vi "EG_G5210 CheckStatus.vi"(6 "ShowStatMess":bool=TRUE caption="Show Status Message", 7 "StatusByteRef":refnum<vi>, 8 "error in (no error)":errorcluster, 9 "Ask Correction":bool, 10 "Autoscale":bool, 11 "Ressource VISA In":refnum<visa-resource-name>="GPIB0::8::INSTR") -> (0 "error out":errorcluster, 1 "Warning":bool, 2 "Ask Correction Out":bool, 3 "Ressource VISA Out":refnum<visa-resource-name>="GPIB0::8::INSTR", 4 "Reprise":bool, 5 "Status Byte":bool[](array[boolean]))   [LabVIEW 2019]
uses:
  <userlib>/EG_G 5210 LIA/CheckStatusState.ctl
  <userlib>/GenProg/WritebyWeakRefNum.vi
panel:
  # "Command Complete"
  # "Command Par Error"
  # "Pll unlck"
  # "New Val Avail"
  # "SRQ Asserted"
  # "Data Available"
  # "Invalid Command"
  # "Overload"
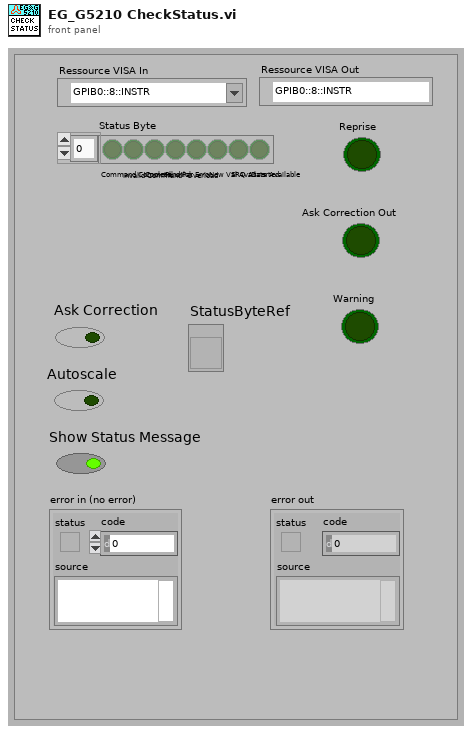
[diagram p1: front panel]
types:
  T1 = typedef "CheckStatusState.ctl" = enum16{"Read Status", "Status Message", "Find Error", "PLL", "Overload", "Change Scale"}
  T2 = enum32{"Invalid", "Standard", "Closed", "Hidden", "Minimized", "Maximized"}
  T3 = enum16{"Left Button", "Center Button", "Right Button", "Window Close"}
  T4 = enum32{"Bad", "Idle", "Run top level", "Running"}
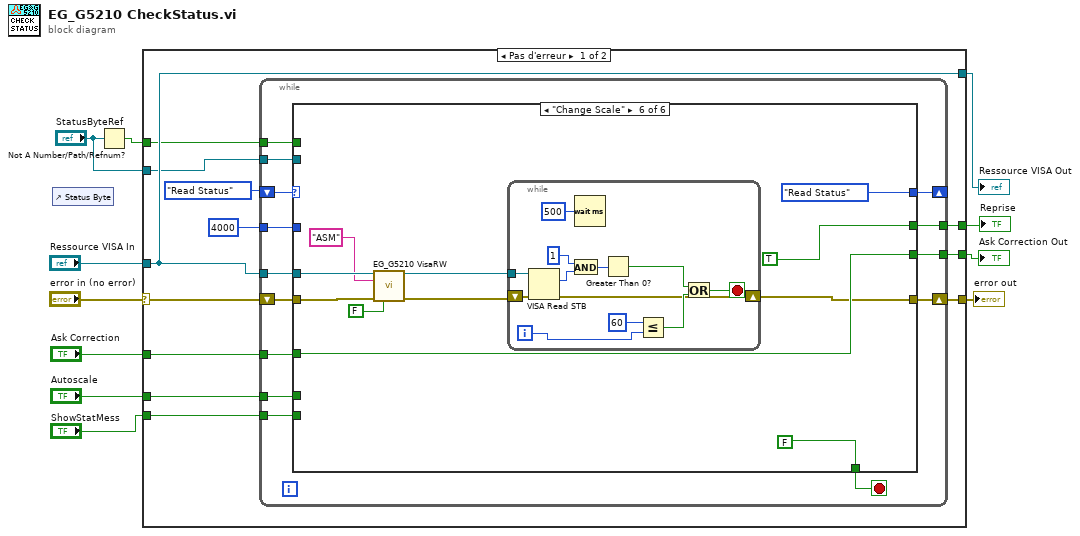
[diagram p0: block diagram]
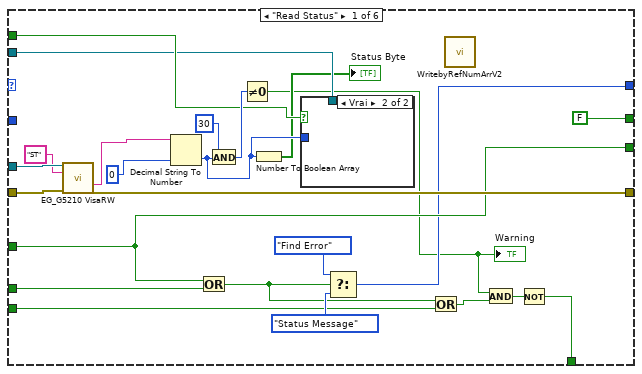
[diagram p2: hidden frame]
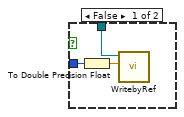
[diagram p3: hidden frame]
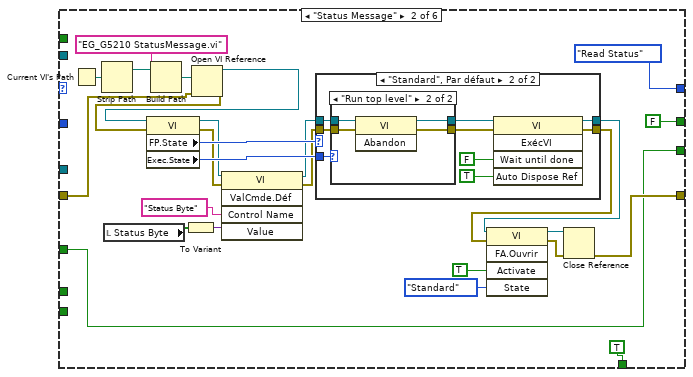
[diagram p4: hidden frame]
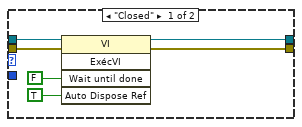
[diagram p5: hidden frame]
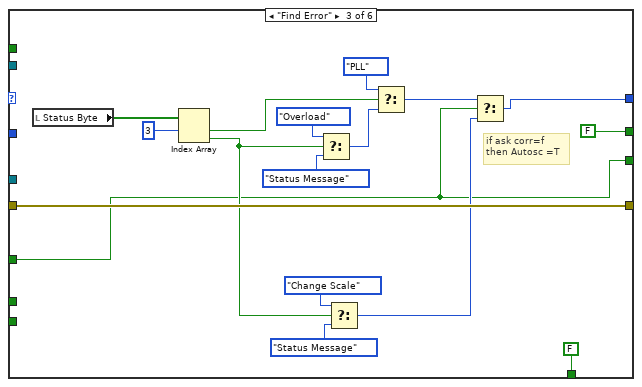
[diagram p7: hidden frame]
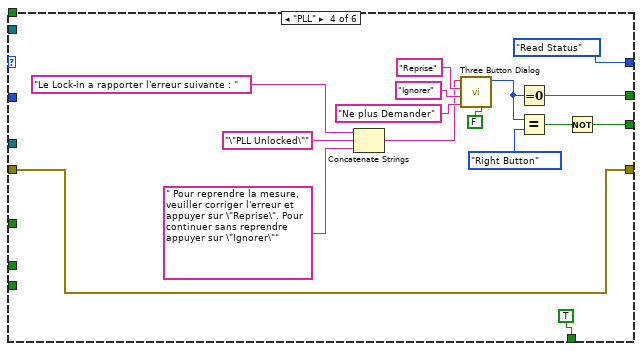
[diagram p8: hidden frame]
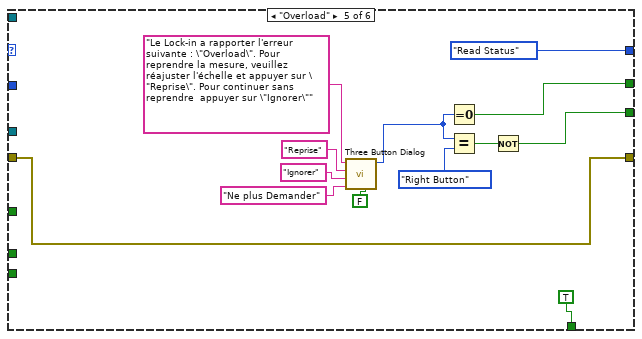
[diagram p9: hidden frame]
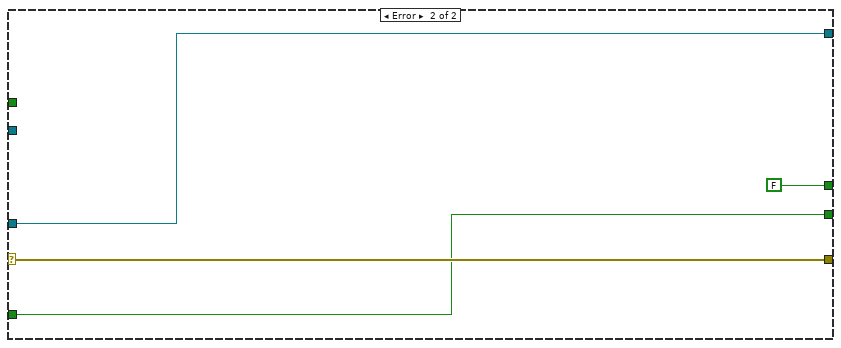
[diagram p10: hidden frame]
diagram:
  n1 = control-ref of="Status Byte"() -> ()  [unwired: 1 out]
  n2 = Not A Number/Path/Refnum?(number/path/refnum="StatusByteRef") -> (NaN/Path/Refnum?=w3:bool)
  n3 = case shown="Pas d'erreur" "error in (no error)" {
    selector: "error in (no error)" -> [w19 w185]
    tunnel: [w22 w185] -> w10
    tunnel: "Autoscale" -> [w21 _]
    tunnel: "Ask Correction" -> [w20 w183]
    tunnel: [w18 FALSE] -> w6
    tunnel: [w17 w183] -> w7
    tunnel: "Ressource VISA In" -> [w16 w182]
    tunnel: [w16 w182] -> w4
    tunnel: w3 -> [w14 _]
    tunnel: "StatusByteRef" -> [w13 _]
    tunnel: "ShowStatMess" -> [w12 _]
    frame No Error {
      n4 = while {
        shift-right: [w32] -> _
        shift-left: CheckStatusState."Read Status" ("Énum") -> [w37]
        shift-right: [w35] -> w22
        shift-left: w19 -> [w36]
        tunnel: 4000 ("timeout ms (488.2 global)") -> [w34]
        tunnel: w21 -> [w31]
        tunnel: w20 -> [w30]
        tunnel: w16 -> [w29]
        tunnel: [w28] -> w18
        tunnel: [w27] -> w17
        tunnel: w14 -> [w26]
        tunnel: w13 -> [w25]
        tunnel: w12 -> [w24]
        stop <- w33 stop-if-true
        n5 = case shown="\"Change Scale\"" w37 {
          tunnel: w36 -> [w61 w78 w124 w134 w157 w169]
          tunnel: [w60 w79 w124 w134 w157 w160] -> w35
          tunnel: w34 -> [_ _ _ _ _ _]
          tunnel: [w38 TRUE FALSE TRUE TRUE FALSE] -> w33
          tunnel: [w52 CheckStatusState."Read Status" w118 CheckStatusState."Read Status" CheckStatusState."Read Status" CheckStatusState."Read Status"] -> w32
          tunnel: w31 -> [w53 _ _ _ _ _]
          tunnel: w30 -> [w54 w73 w113 _ _ w168]
          tunnel: w29 -> [w59 _ _ _ _ w166]
          tunnel: [w54 w73 w113 w131 w155 w168] -> w27
          tunnel: [FALSE FALSE FALSE w133 w156 TRUE] -> w28
          tunnel: w26 -> [w47 _ _ _ _ _]
          tunnel: w25 -> [w45 _ _ _ _ _]
          tunnel: w24 -> [w42 _ _ _ _ _]
          frame "Read Status" {
            n6 = call <userlib>:"EG_G5210 VisaRW.vi"("VISA Rsrc"=w59, "ChaineCom"="ST", "error in (no error)"=w61) -> ("ChaineRep"=w51:string, "error out"=w60:errorcluster)  [unwired: 9 in, 2 out]
            n7 = Decimal String To Number(string=w51, default (0L)=u8 0 ("default (0 I32)")) -> (number=w46:u8)  [unwired: 1 in, 1 out]
            n8 = Or(x=w54, y=w53) -> (x .or. y?=w43:bool)
            n9 = And(x=u8 30, y=w46) -> (x .and. y?=w48:u8)
            n10 = Not Equal To 0?(x=w48) -> (x != 0?=w41:bool)
            "Warning" <- w41
            n11 = Number To Boolean Array(number=w46) -> (Boolean array=→"Status Byte":bool[])
            n12 = case shown="Vrai" w47 {
              tunnel: w46 -> [w63 _]
              tunnel: w45 -> [w64 _]
              frame False {
                n13 = To Double Precision Float(number=w63) -> (double precision float=w62:dbl)
                n14 = call-poly <userlib>:"WritebyRef.vi"("Valeur"=w62, "Control Ref"=w64) -> ()  [unwired: 9 in, 1 out]
              }
              frame True {
              }
            }
            n15 = Select(t=CheckStatusState."Find Error", s=w43, f=CheckStatusState."Status Message") -> (s? t:f=w52:T1)
            n16 = Or(x=w43, y=w42) -> (x .or. y?=w40:bool)
            n17 = call <userlib>:"WritebyRefNumArrV2.vi"() -> ()  [unwired: 11 in, 1 out]
            n18 = And(x=w41, y=w40) -> (x .and. y?=w39:bool)
            n19 = Not(x=w39) -> (.not. x?=w38:bool)
          }
          frame "Status Message" {
            n20 = Current VI's Path() -> (path=w89:path)
            n21 = Strip Path(path=w89) -> (stripped path=w90:path)  [unwired: 1 out]
            n22 = local read "Status Byte"() -> (w76:bool[])
            n23 = Build Path(base path=w90, name or relative path="EG_G5210 StatusMessage.vi" ("nom ou chemin relatif")) -> (appended path=w85:path)
            n24 = To Variant(anything=w76) -> (Variant=w82:variant)
            n25 = Open VI Reference(vi path=w85, error in (no error)=w78) -> (vi reference=w86:refnum<vi>, error out=w77:errorcluster)  [unwired: 4 in]
            n26 = property class="VI"(reference=w86, error in=w77) -> (reference out=w66:refnum<vi>, error out=w67:errorcluster, "FP.State"=w87:T2, "Exec.State"=w88:T4)
            n27 = invoke class="VI" method="ValCmde.Déf"(reference=w66, error in=w67, "Control Name"="Status Byte" ("Nom de la commande"), "Value"=w82) -> (reference out=w68:refnum<vi>, error out=w69:errorcluster)  [unwired: 1 in, 3 out]
            n28 = case shown="\"Standard\", Par défaut" w87 {
              tunnel: [w94 w103] -> w70
              tunnel: w68 -> [w95 w101]
              tunnel: w88 -> [_ w102]
              tunnel: w69 -> [w93 w100]
              tunnel: [w92 w98] -> w71
              frame "Closed" {
                n29 = invoke class="VI" method="ExécVI"(reference=w95, error in=w93, "Wait until done"=FALSE ("Attendre la fin"), "Auto Dispose Ref"=TRUE ("Supprimer la référence automatiquement")) -> (reference out=w94:refnum<vi>, error out=w92:errorcluster)  [unwired: 1 in, 3 out]
              }
              frame "Standard", Default {
                n30 = case shown="\"Run top level\"" w102 {
                  tunnel: [w108 w112] -> w104
                  tunnel: w101 -> [w108 w111]
                  tunnel: w100 -> [w107 w110]
                  tunnel: [w107 w109] -> w99
                  frame "Idle", Default {
                  }
                  frame "Run top level" {
                    n31 = invoke class="VI" method="Abandon"(reference=w111, error in=w110) -> (reference out=w112:refnum<vi>, error out=w109:errorcluster)  [unwired: 1 in, 1 out]
                  }
                }
                n32 = invoke class="VI" method="ExécVI"(reference=w104, error in=w99, "Wait until done"=FALSE ("Attendre la fin"), "Auto Dispose Ref"=TRUE ("Supprimer la référence automatiquement")) -> (reference out=w103:refnum<vi>, error out=w98:errorcluster)  [unwired: 1 in, 3 out]
              }
            }
            n33 = invoke class="VI" method="FA.Ouvrir"(reference=w70, error in=w71, "Activate"=TRUE ("Activer ?"), "State"=T2."Standard" ("État")) -> (reference out=w81:refnum<vi>, error out=w80:errorcluster)  [unwired: 1 in, 3 out]
            n34 = Close Reference(reference=w81, error in (no error)=w80) -> (error out=w79:errorcluster)
          }
          frame "Find Error" {
            # "if ask corr=f\nthen Autosc =T"
            n35 = local read "Status Byte"() -> (w128:bool[])
            n36 = Index Array(array=w128, index #1=3 ("indice")) -> (element #1=w115:bool, element #2=w114:bool)  [unwired: 1 in]
            n37 = Select(t=CheckStatusState."Overload", s=w114, f=CheckStatusState."Status Message") -> (s? t:f=w127:T1)
            n38 = Select(t=CheckStatusState."Change Scale", s=w114, f=CheckStatusState."Status Message") -> (s? t:f=w119:T1)
            n39 = Select(t=CheckStatusState."PLL", s=w115, f=w127) -> (s? t:f=w121:T1)
            n40 = Select(t=w121, s=w113, f=w119) -> (s? t:f=w118:T1)
          }
          frame "PLL" {
            n41 = Concatenate Strings("Le Lock-in a rapporter l'erreur suivante : ", "\"PLL Unlocked\"", " Pour reprendre la mesure, veuiller corriger l'erreur et appuyer sur \"Reprise\". Pour continuer sans reprendre  appuyer sur \"Ignorer\"" ("message")) -> (w139:string)
            n42 = call <vilib>:"Three Button Dialog.vi"("Allow user to close window? (TRUE)"=FALSE, "Right Button Text (\"Cancel\")"="Ne plus Demander" ("F button name (\"Cancel\")"), "Center Button Text (\"No\")"="Ignorer" ("F button name (\"Cancel\")"), "Left Button Text (\"Yes\")"="Reprise" ("T button name (\"OK\")"), "message"=w139) -> ("Which Button?"=w137:T3)  [unwired: 6 in]
            n43 = Equal To 0?(x=w137) -> (x = 0?=w133:bool)
            n44 = Equal?(x=w137, y=T3."Right Button") -> (x = y?=w132:bool)
            n45 = Not(x=w132) -> (.not. x?=w131:bool)
          }
          frame "Overload" {
            n46 = call <vilib>:"Three Button Dialog.vi"("Allow user to close window? (TRUE)"=FALSE, "Right Button Text (\"Cancel\")"="Ne plus Demander" ("F button name (\"Cancel\")"), "Center Button Text (\"No\")"="Ignorer" ("F button name (\"Cancel\")"), "Left Button Text (\"Yes\")"="Reprise" ("T button name (\"OK\")"), "message"="Le Lock-in a rapporter l'erreur suivante : \"Overload\". Pour reprendre la mesure, veuillez réajuster l'échelle et appuyer sur \"Reprise\". Pour continuer sans reprendre  appuyer sur \"Ignorer\"") -> ("Which Button?"=w147:T3)  [unwired: 6 in]
            n47 = Equal To 0?(x=w147) -> (x = 0?=w156:bool)
            n48 = Equal?(x=w147, y=T3."Right Button") -> (x = y?=w146:bool)
            n49 = Not(x=w146) -> (.not. x?=w155:bool)
          }
          frame "Change Scale" {
            n50 = call <userlib>:"EG_G5210 VisaRW.vi"("VISA Rsrc"=w166, "ChaineCom"="ASM", "error in (no error)"=w169, "Lecture?(T)"=FALSE) -> ("VISA Rsrc Out"=w162:refnum<visa-resource-name>, "error out"=w159:errorcluster)  [unwired: 8 in, 2 out]
            n51 = while {
              tunnel: w162 -> [w177]
              shift-right: [w171] -> w160
              shift-left: w159 -> [w170]
              i -> [w180]
              stop <- w178 stop-if-true
              n52 = VISA Read STB(8:w170, 11:w177) -> (0:w171:errorcluster, 2:w176:u16)  [unwired: 1 out]
              n53 = And(x=u16 1, y=w176) -> (x .and. y?=w174:u16)
              n54 = Wait (ms)(milliseconds to wait=u32 500 ("attente (ms)")) -> ()  [unwired: 1 out]
              n55 = Greater Than 0?(x=w174) -> (x > 0?=w172:bool)
              n56 = Less Or Equal?(x=60, y=w180) -> (x <= y?=w173:bool)
              n57 = Or(x=w172, y=w173) -> (x .or. y?=w178:bool)
            }
          }
        }
      }
    }
    frame Error {
    }
  }
  "error out" <- w10
  "Reprise" <- w6
  "Ask Correction Out" <- w7
  "Ressource VISA Out" <- w4
